vi "Json Array example.vi"   [LabVIEW 2017]
uses:
  <vilib>/LVH/i3 JSON/JSON Parsing/Get Object Parameter Files/Get Object Parameter - String.vi
  <vilib>/LVH/i3 JSON/JSON Parsing/Get Object Parameter Files/Get Object Parameter - Object.vi
  <vilib>/LVH/i3 JSON/i3-json.lvlib
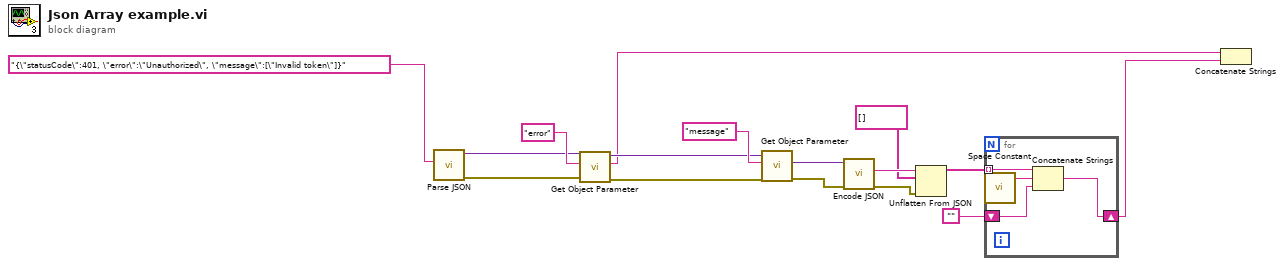
[diagram p0: block diagram]
diagram:
  n1 = call <vilib>:"Parse JSON.vi"("JSON String"="{\"statusCode\":401, \"error\":\"Unauthorized\", \"message\":[\"Invalid token\"]}") -> ("error out"=w6:errorcluster, "JSON Tree"=w5:variant)  [unwired: 7 in, 2 out]
  n2 = call-poly <vilib>:"Get Object Parameter.vi"("error in (no error)"=w6, "Parameter Name"="error", "JSON Tree In (JSON Object)"=w5) -> ("error out"=w3:errorcluster, "String Value"=w2:string, "JSON Tree Out Passthrough"=w4:variant)  [unwired: 5 in, 1 out]
  n3 = call-poly <vilib>:"Get Object Parameter.vi"("error in (no error)"=w3, "Parameter Name"="message", "JSON Tree In (JSON Object)"=w4) -> ("error out"=w14:errorcluster, "JSON Object"=w15:variant)  [unwired: 5 in, 2 out]
  n4 = call <vilib>:"Encode JSON.vi"("error in (no error)"=w14, "JSON Tree"=w15) -> ("error out"=w12:errorcluster, "String"=w13:string)  [unwired: 4 in]
  n5 = Unflatten From JSON(JSON string=w13, type and defaults=string[] [], error in (no error)=w12) -> (value=w9:string[])  [unwired: 4 in, 1 out]
  n6 = for {
    tunnel: w9 -> [w20] mode=indexing
    shift-right: [w17] -> w1
    shift-left: "" -> [w18]
    n7 = call <vilib>:"Space Constant.vi"() -> ("String"=w19:string)
    n8 = Concatenate Strings(w20, w19, w18) -> (w17:string)
  }
  n9 = Concatenate Strings(w2, w1) -> ()  [unwired: 1 out]
